vi "ReadFile.vi"(9 "error in":errorcluster, 11 "Path":path) -> (0 "error out":errorcluster, 1 "size":i32, 2 "Value Array":string[](array[string]), 3 "Value OUT":string)   [LabVIEW 2017]
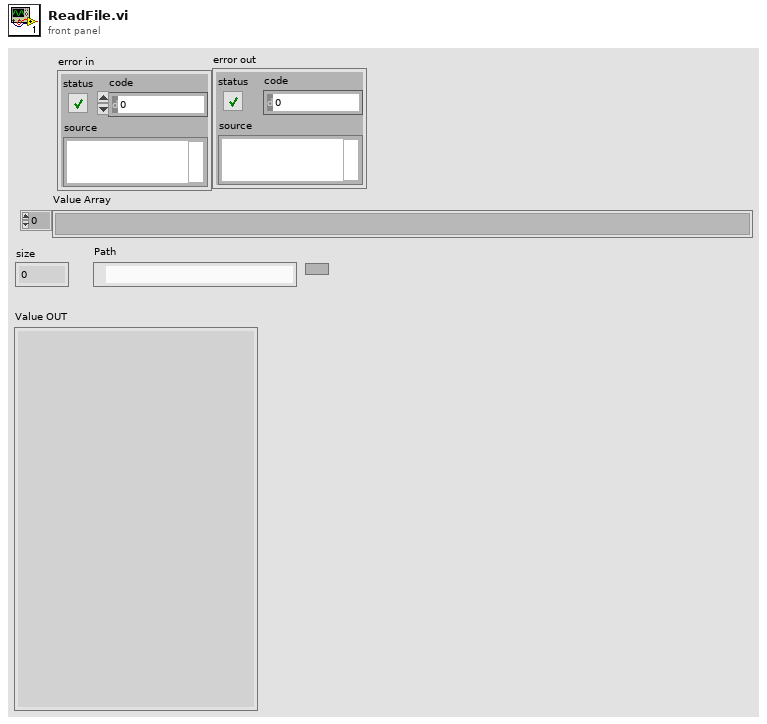
[diagram p1: front panel]
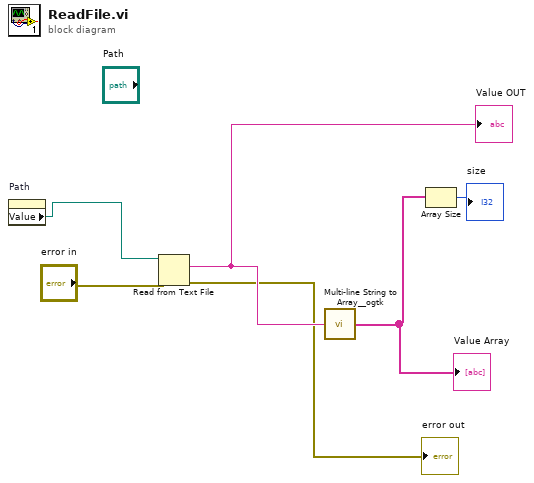
[diagram p0: block diagram]
diagram:
  n1 = property on="Path" class="Path"() -> ("Value"=w1:path)  [unwired: 2 in, 2 out]
  n2 = Read from Text File(file (use dialog)=w1, error in="error in") -> (text=w6:string, error out=→"error out":errorcluster)  [unwired: 2 in, 2 out]
  "Value OUT" <- w6
  n3 = call "Multi-line String to Array__ogtk.vi"("string"=w6) -> ("lines"=w5:string[])
  "Value Array" <- w5
  n4 = Array Size(array=w5) -> (size(s)=→"size":i32)
